vi "ReadContinous.vi"(8 "error in (no error)":errorcluster, 9 "Max samples to keep":u32, 10 "Min samples to read":u32, 11 "Scope5785_six_channel":refnum<class "Scope5782_six_channel.lvclass">) -> (0 "error out":errorcluster, 1 "#elements":i32, 2 "Data":dbl[][](array[numeric]), 3 "Scope5785_six_channel Out":refnum<class "Scope5782_six_channel.lvclass">)   [LabVIEW 2018, in "Scope5782_six_channel.lvclass"]
uses:
  Scope5782_six_channel.lvclass
  C:/PXIe/InProgress/source2/Host/Scope/ScopeBase/ScopeBase.lvclass
  controls/host_transfer_speed.ctl
  ScopeBase/ScopeBase.lvclass/ScopeBase.ctl
  Scope5782_six_channel.lvclass/Scope5782_six_channel.ctl
  FpgaRef/FpgaRef5761/FpgaRef5761.lvclass
  FpgaRef/FpgaRef5782/FpgaRef5782.lvclass
  ScopeBase/ScopeBase.lvclass
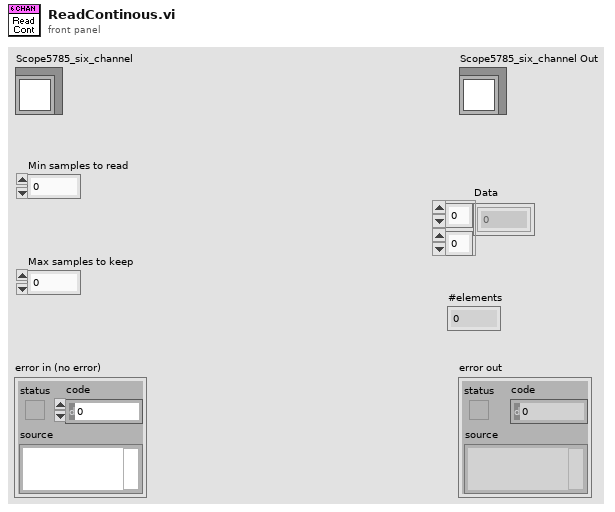
[diagram p1: front panel]
types:
  T1 = typedef "host_transfer_speed.ctl" = enum16{"Very high speed (10Ms/s)", "High speed (1Ms/s)", "Low speed (50kS/s)", "Ultra low speed (20kS/s)"}
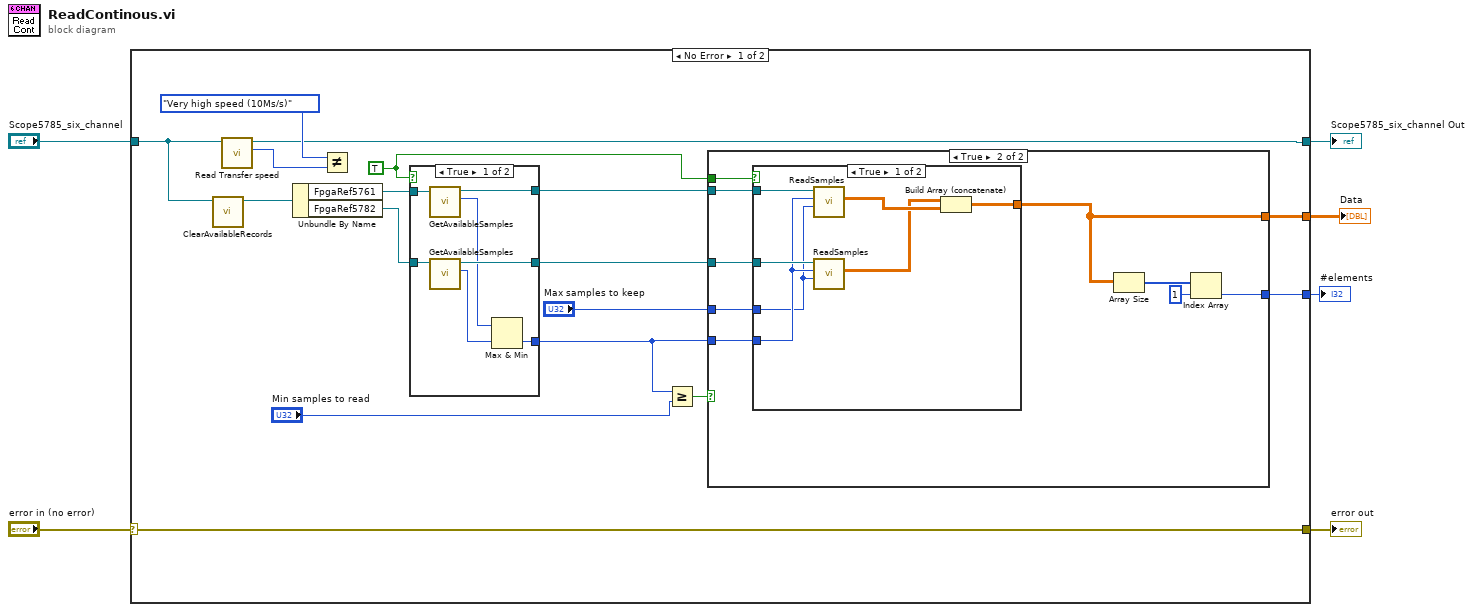
[diagram p0: block diagram]
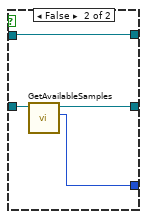
[diagram p2: hidden frame]
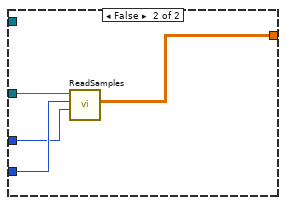
[diagram p4: hidden frame]
diagram:
  n1 = case shown="No Error" "error in (no error)" {
    selector: "error in (no error)" -> [w23 w56]
    tunnel: [w23 w56] -> w5
    tunnel: [w8 w55] -> w3
    tunnel: "Scope5785_six_channel" -> [w9 w55]
    tunnel: [w22 _] -> w2
    tunnel: [w21 _] -> w1
    frame No Error {
      w7 = TRUE ("x != y?")
      n2 = call "ClearAvailableRecords.vi"("Scope5785_six_channel"=w9) -> ("Scope5785_six_channel out"=w20:refnum<class "Scope5782_six_channel.lvclass">)  [unwired: 9 in, 1 out]
      n3 = call "Read Transfer speed.vi"("ScopeBase in"=w9) -> ("Tranfer speed"=w11:T1, "ScopeBase out"=w8:refnum<class "Scope5782_six_channel.lvclass">)  [unwired: 8 in, 1 out]
      n4 = Unbundle By Name(w20) -> ("FpgaRef5761"=w19:refnum<class "FpgaRef5761.lvclass">, "FpgaRef5782"=w18:refnum<class "FpgaRef5782.lvclass">)
      n5 = Not Equal?(x=host_transfer_speed."Very high speed (10Ms/s)" ("y"), y=w11) -> ()  [unwired: 1 out]
      n6 = case shown="True" w7 {
        tunnel: w19 -> [w30 w31]
        tunnel: w18 -> [w29 w34]
        tunnel: [w27 w32] -> w15
        tunnel: [w26 w31] -> w13
        tunnel: [w25 w33] -> w12
        frame True {
          n7 = call-dynamic "GetAvailableSamples.vi"("FpgaRef5761 In"=w30) -> ("available"=w24:u32, "FpgaRef5761 Out"=w26:refnum<class "FpgaRef5761.lvclass">)  [unwired: 8 in, 1 out]
          n8 = call-dynamic "GetAvailableSamples.vi"("FpgaRef5782 in"=w29) -> ("available"=w28:u32, "FpgaRef5782 out"=w25:refnum<class "FpgaRef5782.lvclass">)  [unwired: 8 in, 1 out]
          n9 = Max & Min(x=w24, y=w28) -> (min(x,y)=w27:u32)  [unwired: 1 out]
        }
        frame False {
          n10 = call-dynamic "GetAvailableSamples.vi"("FpgaRef5782 in"=w34) -> ("available"=w32:u32, "FpgaRef5782 out"=w33:refnum<class "FpgaRef5782.lvclass">)  [unwired: 8 in, 1 out]
        }
      }
      n11 = Greater Or Equal?(x=w15, y="Min samples to read") -> (x >= y?=w16:bool)
      n12 = case shown="True" w16 {
        tunnel: [_ w43] -> w22
        tunnel: [_ w40] -> w21
        tunnel: w15 -> [_ w37]
        tunnel: "Max samples to keep" -> [_ w36]
        tunnel: w13 -> [_ w39]
        tunnel: w12 -> [_ w38]
        tunnel: w7 -> [_ w35]
        frame False {
        }
        frame True {
          n13 = case shown="True" w35 {
            tunnel: [w50 w51] -> w43
            tunnel: w39 -> [w49 _]
            tunnel: w38 -> [w48 w54]
            tunnel: w37 -> [w47 w53]
            tunnel: w36 -> [w44 w52]
            frame True {
              n14 = call-dynamic "ReadSamples.vi"("Max num samples to keep"=w44, "Num samples to read"=w47, "FpgaRef5761 In"=w49) -> ("Data"=w46:dbl[][])  [unwired: 6 in, 2 out]
              n15 = call-dynamic "ReadSamples.vi"("Max num samples to keep"=w44, "Num samples to read"=w47, "FpgaRef5782 in"=w48) -> ("Data"=w45:dbl[][])  [unwired: 6 in, 2 out]
              n16 = Build Array (concatenate)(w45, w46) -> (w50:dbl[][])
            }
            frame False {
              n17 = call-dynamic "ReadSamples.vi"("Max num samples to keep"=w52, "Num samples to read"=w53, "FpgaRef5782 in"=w54) -> ("Data"=w51:dbl[][])  [unwired: 6 in, 2 out]
            }
          }
          n18 = Array Size(array=w43) -> (size(s)=w42:i32[])
          n19 = Index Array(array=w42, index=1) -> (element=w40:i32)
        }
      }
    }
    frame Error {
    }
  }
  "error out" <- w5
  "Scope5785_six_channel Out" <- w3
  "Data" <- w2
  "#elements" <- w1
